vi "Write Language.vi"(8 "error in (no error)":errorcluster, 10 "Language":T1, 11 "Prooduct Actor in":refnum<class "Prooduct Actor.lvclass">) -> (0 "error out":errorcluster, 3 "Prooduct Actor out":refnum<class "Prooduct Actor.lvclass">)   [LabVIEW 2020, in "Prooduct Actor.lvlib" / "Prooduct Actor.lvclass"]
uses:
  Prooduct Actor.lvclass
  Controls/Language Enum.ctl
  Prooduct Actor.lvclass/Prooduct Actor.ctl
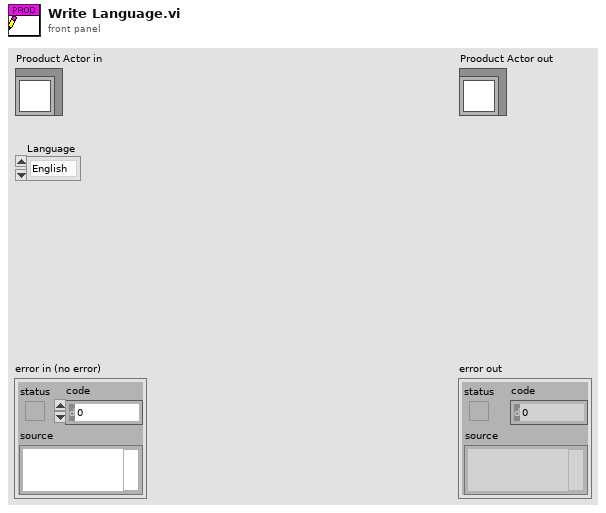
[diagram p1: front panel]
types:
  T1 = typedef "Language Enum.ctl" = enum16{"English", "Español", "Français"}
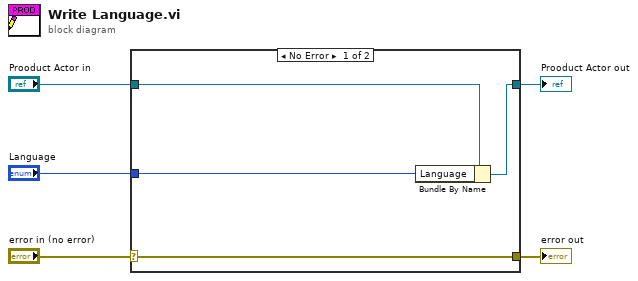
[diagram p0: block diagram]
diagram:
  n1 = case shown="No Error" "error in (no error)" {
    selector: "error in (no error)" -> [w9 w10]
    tunnel: [w9 w10] -> w4
    tunnel: [w7 w11] -> w2
    tunnel: "Prooduct Actor in" -> [w8 w11]
    tunnel: "Language" -> [w6 _]
    frame No Error {
      n2 = Bundle By Name(cluster=w8, "Language"=w6) -> (w7:refnum<class "Prooduct Actor.lvclass">)
    }
    frame Error {
    }
  }
  "error out" <- w4
  "Prooduct Actor out" <- w2
